vi "Test pinMode.vi"(8 "Error In":errorcluster, 10 "Pin number":u8, 11 "Pin mode":u8) -> (0 "Error Out":errorcluster)   [LabVIEW 2014, in "STM32F4 Discovery General Wrapper.lvlib"]
uses:
  <vilib>/Aledyne-TSXperts/Arduino Compatible Compiler for LabVIEW/addons/STM32F4 Discovery General Wrapper/STM32F4 Discovery General Wrapper.lvlib
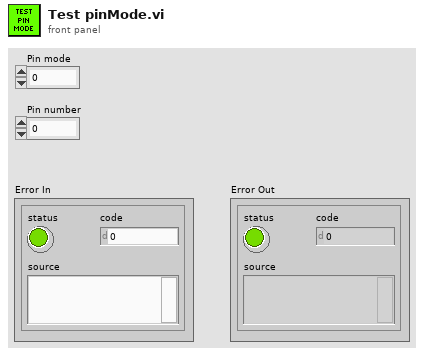
[diagram p1: front panel]
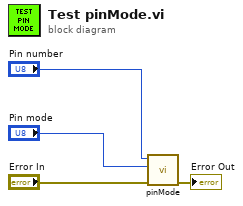
[diagram p0: block diagram]
diagram:
  n1 = call <vilib>:"pinMode.vi"("Error In"="Error In", "Pin mode"="Pin mode", "Pin number"="Pin number") -> ("Error Out"=→"Error Out":errorcluster)  [unwired: 8 in]
